vi "String - Convert MAC Address Hexidecimal Array to String.vi"(11 "Hexidecimal Strings":string[](array[string])) -> (3 "MAC Address String":string)   [LabVIEW 2020]
doc: "Converts an array of hexidecimal string into a MAC address string."
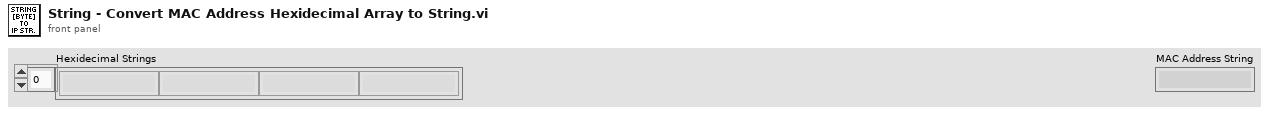
[diagram p1: front panel]
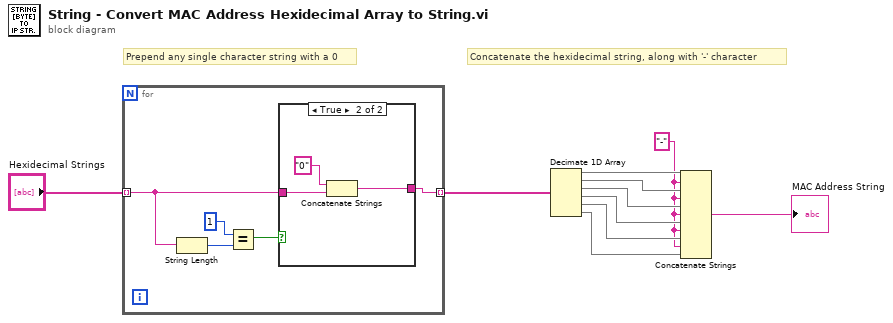
[diagram p0: block diagram]
diagram:
  w4 = "-"
  # "Prepend any single character string with a 0"
  # "Concatenate the hexidecimal string, along with '-' character"
  n1 = for {
    tunnel: "Hexidecimal Strings" -> [w12] mode=indexing
    tunnel: [w11] -> w1 mode=indexing
    n2 = String Length(string=w12) -> (length=w15:i32)
    n3 = Equal?(x=1, y=w15) -> (x = y?=w13:bool)
    n4 = case shown="True" w13 {
      tunnel: w12 -> [w16 w19]
      tunnel: [w16 w17] -> w11
      frame False {
      }
      frame True {
        n5 = Concatenate Strings("0" ("string"), w19) -> (w17:string)
      }
    }
  }
  n6 = Decimate 1D Array(w1) -> (w6:string[], w7:string[], w8:string[], w9:string[], w5:string[], w3:string[])
  n7 = Concatenate Strings(w6, w4, w7, w4, w8, w4, w9, w4, w5, w4, w3) -> (→"MAC Address String":string)
